vi "E7_28_readstring.vi"(5 "read buffer":string) -> (1 "Offset":dbl, 2 "Level":dbl, 3 "Frequency":dbl, 4 "FLAGS":dbl, 6 "ImParam_Value":dbl, 8 "Mode":dbl, 10 "SecParam_Value":dbl, 12 "OnChange":dbl, 13 "SecParam":dbl, 14 "ImParam":dbl, 15 "Limit":dbl)   [LabVIEW 2018]
panel:
  out "CS":dbl
  out "substring":string
  out "after substring":string
  out "before substring":string
  out "0xAA":string
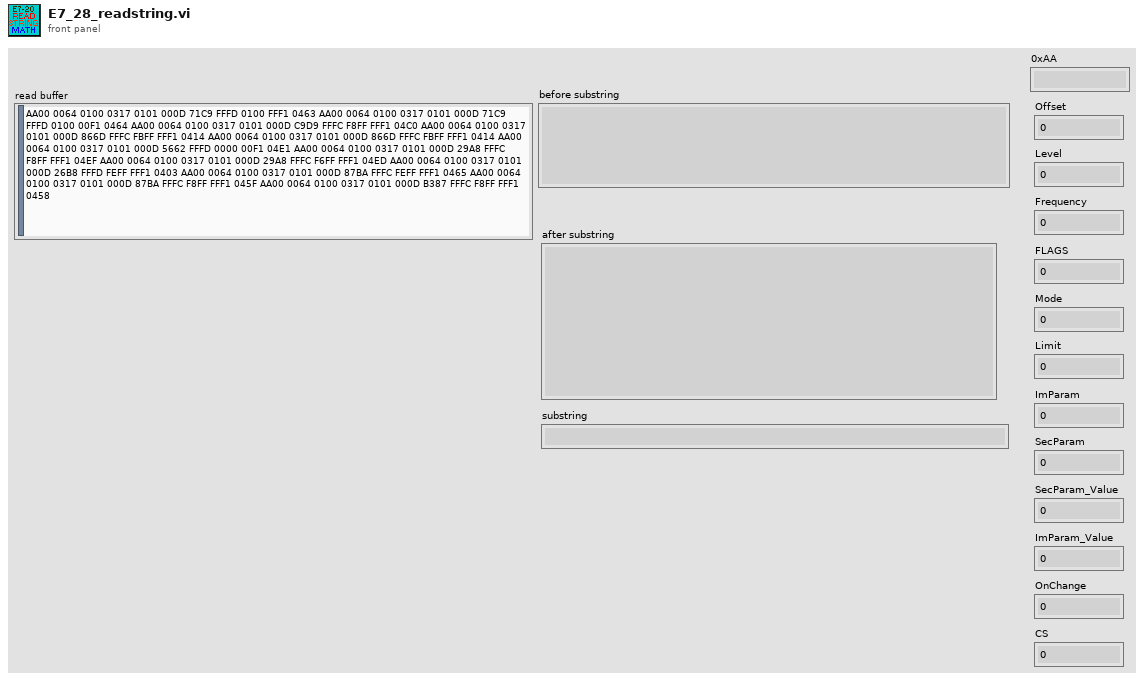
[diagram p1: front panel]
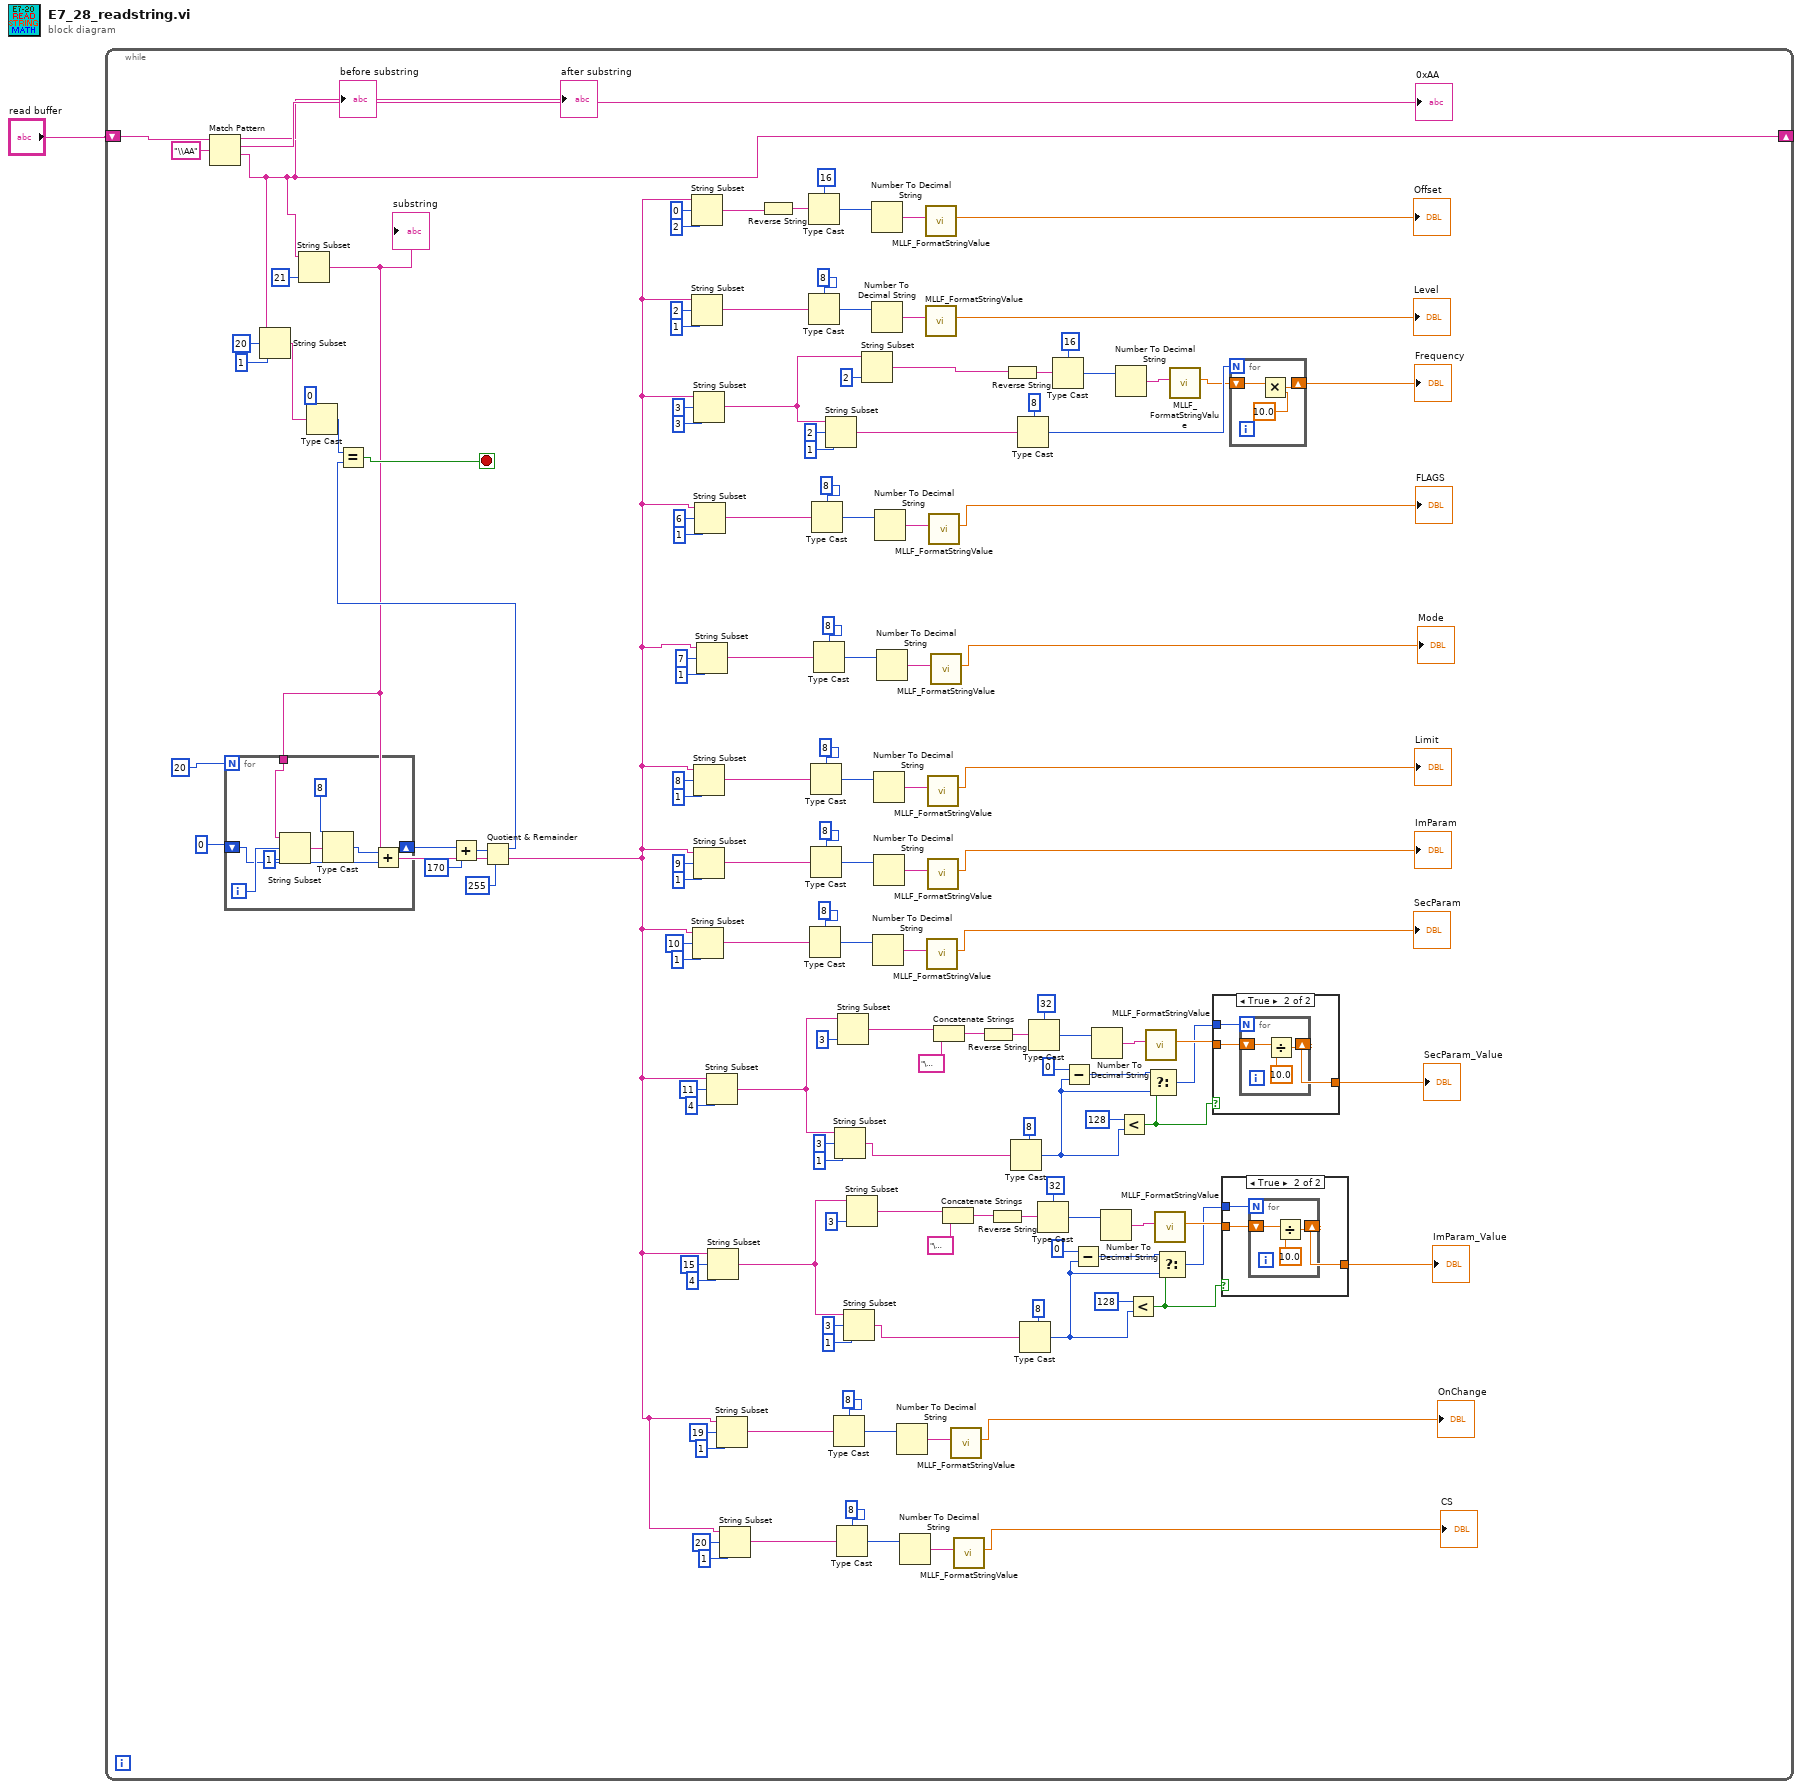
[diagram p0: block diagram]
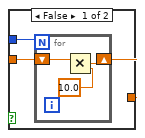
[diagram p2: hidden frame]
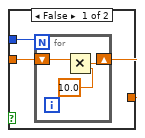
[diagram p3: hidden frame]
diagram:
  n1 = while {
    shift-right: [w124] -> _
    shift-left: "read buffer" -> [w125]
    stop <- w52 stop-if-true
    n2 = Match Pattern(string=w125, regular expression="\\AA") -> (before substring=→"before substring":string, match substring=→"0xAA":string, after substring=w124:string)  [unwired: 1 in, 1 out]
    "after substring" <- w124
    n3 = String Subset(string=w124, offset (0)=20, length (rest)=1 ("length (rest)")) -> (substring=w127:string)
    n4 = String Subset(string=w124, length (rest)=21 ("length (rest)")) -> (substring=w2:string)  [unwired: 1 in]
    "substring" <- w2
    n5 = for {
      N: 20 ("length (rest)") -> [_]
      tunnel: w2 -> [w149]
      shift-right: [w150] -> w71
      shift-left: u8 0 -> [w151]
      i -> [w154]
      n6 = String Subset(string=w149, offset (0)=w154, length (rest)=1 ("length (rest)")) -> (substring=w152:string)
      n7 = Type Cast(type=u8 8, x=w152) -> (*(type *) &x=w148:u8)
      n8 = Add(x=w148, y=w151) -> (x+y=w150:u8)
    }
    n9 = Type Cast(type=u8 0, x=w127) -> (*(type *) &x=w126:u8)
    n10 = Add(x=w71, y=u8 170 ("length (rest)")) -> (x+y=w70:u8)
    n11 = Quotient & Remainder(x=w70, y=u8 255 ("length (rest)")) -> (x-y*floor(x/y)=w53:u8)  [unwired: 1 out]
    n12 = Equal?(x=w126, y=w53) -> (x = y?=w52:bool)
    n13 = String Subset(string=w2, offset (0)=0 ("length (rest)"), length (rest)=2 ("length (rest)")) -> (substring=w86:string)
    n14 = String Subset(string=w2, offset (0)=2 ("length (rest)"), length (rest)=1 ("length (rest)")) -> (substring=w78:string)
    n15 = String Subset(string=w2, offset (0)=10 ("length (rest)"), length (rest)=1 ("length (rest)")) -> (substring=w22:string)
    n16 = String Subset(string=w2, offset (0)=3 ("length (rest)"), length (rest)=3 ("length (rest)")) -> (substring=w56:string)
    n17 = String Subset(string=w2, offset (0)=8 ("length (rest)"), length (rest)=1 ("length (rest)")) -> (substring=w32:string)
    n18 = String Subset(string=w2, offset (0)=9 ("length (rest)"), length (rest)=1 ("length (rest)")) -> (substring=w29:string)
    n19 = String Subset(string=w2, offset (0)=6 ("length (rest)"), length (rest)=1 ("length (rest)")) -> (substring=w46:string)
    n20 = String Subset(string=w2, offset (0)=7 ("length (rest)"), length (rest)=1 ("length (rest)")) -> (substring=w39:string)
    n21 = String Subset(string=w2, offset (0)=11 ("length (rest)"), length (rest)=4 ("length (rest)")) -> (substring=w93:string)
    n22 = String Subset(string=w2, offset (0)=15 ("length (rest)"), length (rest)=4 ("length (rest)")) -> (substring=w140:string)
    n23 = String Subset(string=w2, offset (0)=19 ("length (rest)"), length (rest)=1 ("length (rest)")) -> (substring=w15:string)
    n24 = String Subset(string=w2, offset (0)=20 ("length (rest)"), length (rest)=1 ("length (rest)")) -> (substring=w8:string)
    n25 = Reverse String(1:w86) -> (0:w88:string)
    n26 = Type Cast(type=u16 16, x=w88) -> (*(type *) &x=w89:u16)
    n27 = Type Cast(type=u8 8, x=w78) -> (*(type *) &x=w80:u8)
    n28 = Type Cast(type=u8 8, x=w22) -> (*(type *) &x=w20:u8)
    n29 = Type Cast(type=u8 8, x=w32) -> (*(type *) &x=w34:u8)
    n30 = Type Cast(type=u8 8, x=w29) -> (*(type *) &x=w27:u8)
    n31 = Type Cast(type=u8 8, x=w46) -> (*(type *) &x=w48:u8)
    n32 = Type Cast(type=u8 8, x=w39) -> (*(type *) &x=w41:u8)
    n33 = String Subset(string=w56, offset (0)=2, length (rest)=1 ("length (rest)")) -> (substring=w65:string)
    n34 = Type Cast(type=u8 8, x=w15) -> (*(type *) &x=w13:u8)
    n35 = String Subset(string=w93, offset (0)=3, length (rest)=1 ("length (rest)")) -> (substring=w110:string)
    n36 = Type Cast(type=u8 8, x=w8) -> (*(type *) &x=w6:u8)
    n37 = String Subset(string=w93, length (rest)=3 ("length (rest)")) -> (substring=w62:string)  [unwired: 1 in]
    n38 = String Subset(string=w140, offset (0)=3, length (rest)=1 ("length (rest)")) -> (substring=w137:string)
    n39 = String Subset(string=w140, length (rest)=3 ("length (rest)")) -> (substring=w133:string)  [unwired: 1 in]
    n40 = String Subset(string=w56, length (rest)=2 ("length (rest)")) -> (substring=w54:string)  [unwired: 1 in]
    n41 = Number To Decimal String(number=w89) -> (decimal integer string=w87:string)  [unwired: 1 in]
    n42 = Number To Decimal String(number=w80) -> (decimal integer string=w82:string)  [unwired: 1 in]
    n43 = Number To Decimal String(number=w20) -> (decimal integer string=w19:string)  [unwired: 1 in]
    n44 = Number To Decimal String(number=w34) -> (decimal integer string=w35:string)  [unwired: 1 in]
    n45 = Number To Decimal String(number=w27) -> (decimal integer string=w26:string)  [unwired: 1 in]
    n46 = Number To Decimal String(number=w48) -> (decimal integer string=w49:string)  [unwired: 1 in]
    n47 = Number To Decimal String(number=w41) -> (decimal integer string=w42:string)  [unwired: 1 in]
    n48 = Number To Decimal String(number=w13) -> (decimal integer string=w12:string)  [unwired: 1 in]
    n49 = Number To Decimal String(number=w6) -> (decimal integer string=w5:string)  [unwired: 1 in]
    n50 = call "MLLF_FormatStringValue.vi"("String Value"=w87) -> ("number"=→"Offset":dbl)  [unwired: 8 in, 2 out]
    n51 = call "MLLF_FormatStringValue.vi"("String Value"=w82) -> ("number"=→"Level":dbl)  [unwired: 8 in, 2 out]
    n52 = call "MLLF_FormatStringValue.vi"("String Value"=w19) -> ("number"=→"SecParam":dbl)  [unwired: 8 in, 2 out]
    n53 = call "MLLF_FormatStringValue.vi"("String Value"=w35) -> ("number"=→"Limit":dbl)  [unwired: 8 in, 2 out]
    n54 = call "MLLF_FormatStringValue.vi"("String Value"=w26) -> ("number"=→"ImParam":dbl)  [unwired: 8 in, 2 out]
    n55 = call "MLLF_FormatStringValue.vi"("String Value"=w49) -> ("number"=→"FLAGS":dbl)  [unwired: 8 in, 2 out]
    n56 = call "MLLF_FormatStringValue.vi"("String Value"=w42) -> ("number"=→"Mode":dbl)  [unwired: 8 in, 2 out]
    n57 = Concatenate Strings(w62, "\u0000" ("string")) -> (w106:string)
    n58 = Concatenate Strings(w133, "\u0000" ("string")) -> (w132:string)
    n59 = call "MLLF_FormatStringValue.vi"("String Value"=w12) -> ("number"=→"OnChange":dbl)  [unwired: 8 in, 2 out]
    n60 = call "MLLF_FormatStringValue.vi"("String Value"=w5) -> ("number"=→"CS":dbl)  [unwired: 8 in, 2 out]
    n61 = Reverse String(1:w106) -> (0:w104:string)
    n62 = Reverse String(1:w132) -> (0:w122:string)
    n63 = Reverse String(1:w54) -> (0:w59:string)
    n64 = Type Cast(type=u8 8, x=w110) -> (*(type *) &x=w98:u8)
    n65 = Type Cast(type=u8 8, x=w65) -> (*(type *) &x=w64:u8)
    n66 = Type Cast(type=u8 8, x=w137) -> (*(type *) &x=w116:u8)
    n67 = Type Cast(type=u32 32, x=w104) -> (*(type *) &x=w63:u32)
    n68 = Type Cast(type=u32 32, x=w122) -> (*(type *) &x=w123:u32)
    n69 = Type Cast(type=u16 16, x=w59) -> (*(type *) &x=w57:u16)
    n70 = Subtract(x=u8 0, y=w98) -> (x-y=w100:u8)
    n71 = Subtract(x=u8 0, y=w116) -> (x-y=w118:u8)
    n72 = Number To Decimal String(number=w63) -> (decimal integer string=w103:string)  [unwired: 1 in]
    n73 = Number To Decimal String(number=w123) -> (decimal integer string=w121:string)  [unwired: 1 in]
    n74 = Number To Decimal String(number=w57) -> (decimal integer string=w58:string)  [unwired: 1 in]
    n75 = Less?(x=u8 128, y=w98) -> (x < y?=w97:bool)
    n76 = Less?(x=u8 128, y=w116) -> (x < y?=w115:bool)
    n77 = call "MLLF_FormatStringValue.vi"("String Value"=w103) -> ("number"=w102:dbl)  [unwired: 8 in, 2 out]
    n78 = Select(t=w100, s=w97, f=w98) -> (s? t:f=w96:u8)
    n79 = call "MLLF_FormatStringValue.vi"("String Value"=w121) -> ("number"=w120:dbl)  [unwired: 8 in, 2 out]
    n80 = Select(t=w118, s=w115, f=w116) -> (s? t:f=w114:u8)
    n81 = call "MLLF_FormatStringValue.vi"("String Value"=w58) -> ("number"=w55:dbl)  [unwired: 8 in, 2 out]
    n82 = case shown="True" w97 {
      tunnel: w102 -> [w161 w167]
      tunnel: [w160 w166] -> w101
      tunnel: w96 -> [w159 w165]
      frame False {
        n83 = for {
          N: w159 -> [_]
          shift-right: [w164] -> w160
          shift-left: w161 -> [w162]
          n84 = Multiply(x=w162, y=10.0) -> (x*y=w164:dbl)
        }
      }
      frame True {
        n85 = for {
          N: w165 -> [_]
          shift-right: [w168] -> w166
          shift-left: w167 -> [w170]
          n86 = Divide(x=w170, y=10.0) -> (x/y=w168:dbl)
        }
      }
    }
    "SecParam_Value" <- w101
    n87 = case shown="True" w115 {
      tunnel: w120 -> [w173 w179]
      tunnel: [w172 w178] -> w119
      tunnel: w114 -> [w171 w177]
      frame False {
        n88 = for {
          N: w171 -> [_]
          shift-right: [w176] -> w172
          shift-left: w173 -> [w174]
          n89 = Multiply(x=w174, y=10.0) -> (x*y=w176:dbl)
        }
      }
      frame True {
        n90 = for {
          N: w177 -> [_]
          shift-right: [w180] -> w178
          shift-left: w179 -> [w182]
          n91 = Divide(x=w182, y=10.0) -> (x/y=w180:dbl)
        }
      }
    }
    "ImParam_Value" <- w119
    n92 = for {
      N: w64 -> [_]
      shift-right: [w158] -> w72
      shift-left: w55 -> [w156]
      n93 = Multiply(x=w156, y=10.0) -> (x*y=w158:dbl)
    }
    "Frequency" <- w72
  }
